vi "gugudan server.vi"() -> ()   [LabVIEW 2014]
uses:
  <vilib>/FTP/NI_FTP.lvlib
panel:
  out "불리언":bool
  in  "사용설명서":bool
  out "로그인":bool
  in  "ID":string="ID"
  in  "PW":string="PW"
  in  "명령전달":bool
  in  "address":string="ip address"
  out "명령코드":i16[](array[numeric])
  out "참 거짓":string="상태창입니다."
  out "문자열":string="q 입력시 종료 / r 입력시 종료 취소  숫자 1~3번 은 1~3시간 예약 종료 입니다."
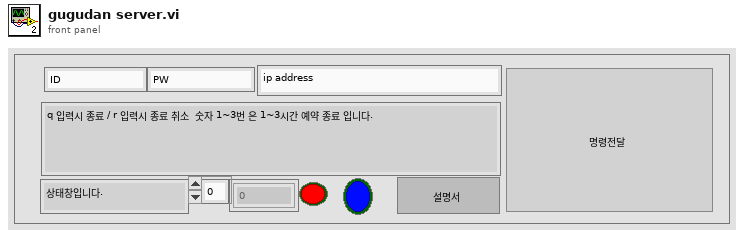
[diagram p1: front panel]
types:
  T1 = typedef "NI_FTP.lvlib/FTP Session.ctl" = refnum<k5>
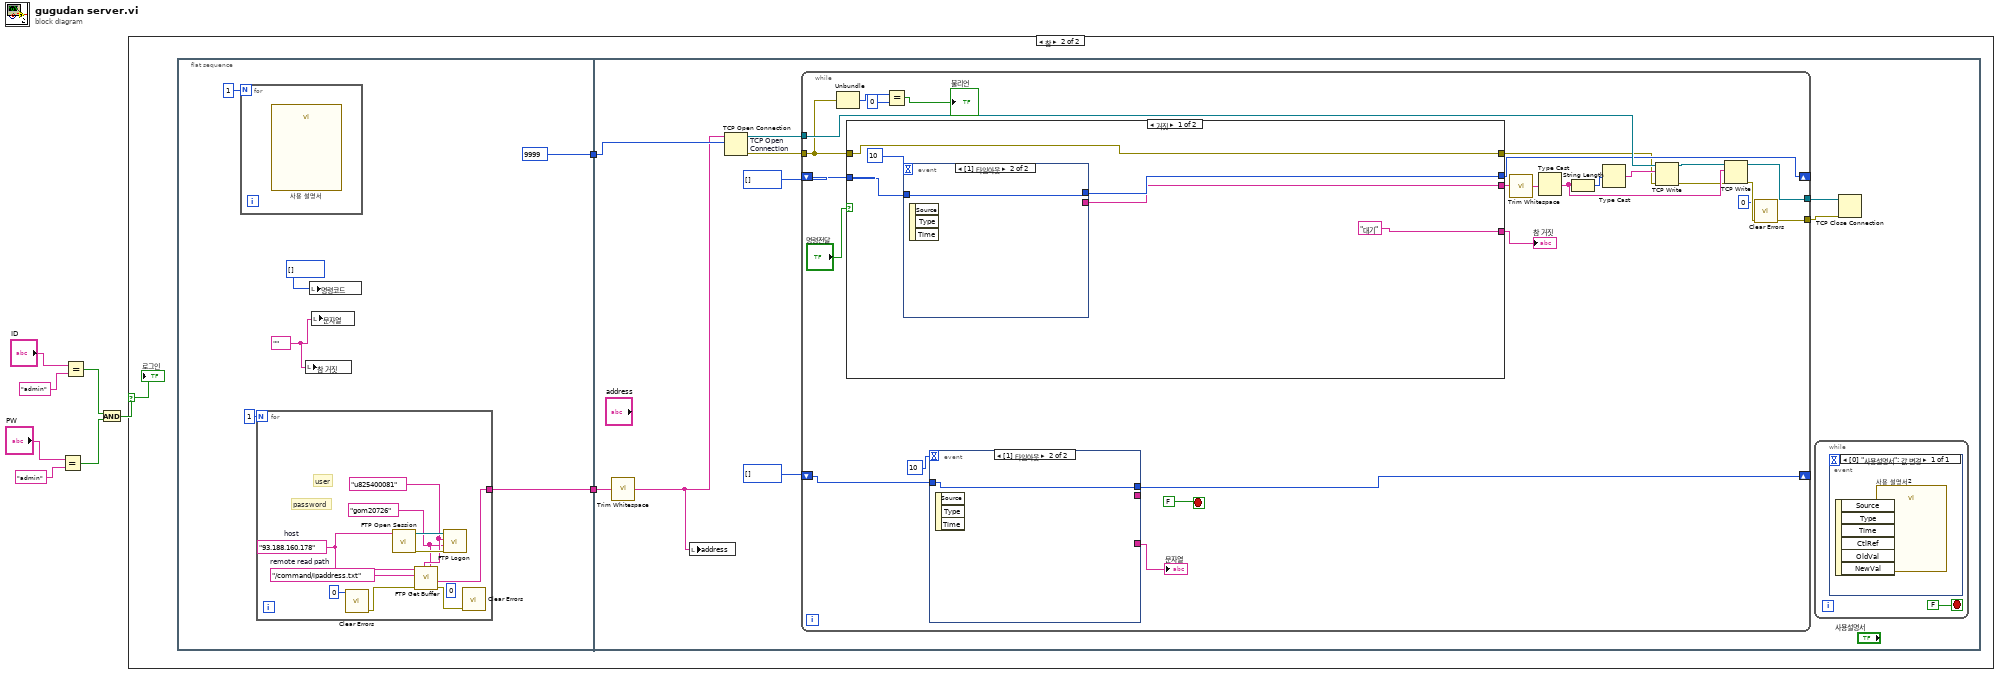
[diagram p0: block diagram]
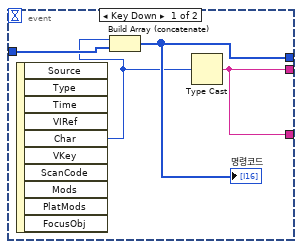
[diagram p3: hidden frame]
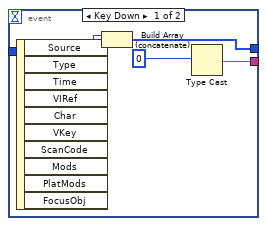
[diagram p4: hidden frame]
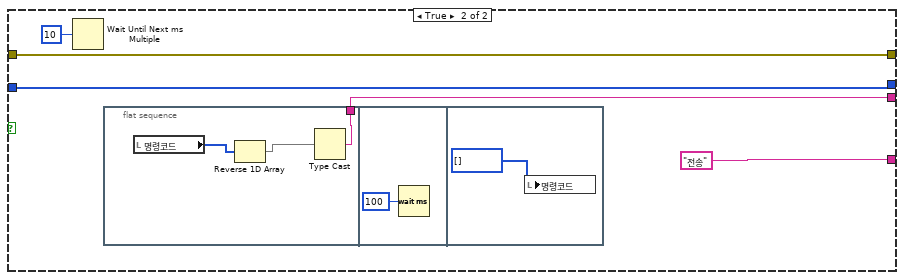
[diagram p5: hidden frame]
diagram:
  n1 = Equal?(x="PW", y="admin") -> (x = y?=w2:bool)
  n2 = Equal?(x="ID", y="admin") -> (x = y?=w3:bool)
  n3 = And(x=w3, y=w2) -> (x .and. y?=w1:bool)
  n4 = case shown="참" w1 {
    selector: w1 -> [_ w10]
    frame False {
    }
    frame True {
      n5 = flat-sequence {
        tunnel: [w12] -> w9
        tunnel: [u16 9999 ("remote port or service name")] -> w8
        tunnel: w9 -> [w29]
        tunnel: w8 -> [w28]
        frame #0 {
          w15 = ""
          n6 = for {
            N: 1 -> [_]
            n7 = call "사용 설명서"() -> ()  [unwired: 10 in, 2 out]
          }
          n8 = for {
            N: 1 -> [_]
            tunnel: [w20] -> w12
            (unwired) 0 ("specific error code to clear (0: all)")
            w23 = "gom20726"
            w24 = "u825400081"
            w21 = "/command/ipaddress.txt"  # remote read path
            w22 = "93.188.160.178"  # host
            # "user"
            # "password"
            n9 = call <vilib>:"Clear Errors.vi"("specific error code to clear (0: all)"=0) -> ("error out"=w19:errorcluster)  [unwired: 5 in, 1 out]
            n10 = call <vilib>:"FTP Open Session.vi"("address"=w22) -> ("error out"=w25:errorcluster, "ftp session"=w26:T1)  [unwired: 7 in, 2 out]
            n11 = call <vilib>:"FTP Get Buffer.vi"("password"=w23, "user"=w24, "error in (no error)"=w19, "remote path"=w21, "host"=w22) -> ("error out"=w17:errorcluster, "data"=w20:string)  [unwired: 4 in, 1 out]
            n12 = call <vilib>:"FTP Logon.vi"("error in (no error)"=w25, "password"=w23, "user"=w24, "ftp session"=w26) -> ()  [unwired: 4 in, 4 out]
            n13 = call <vilib>:"Clear Errors.vi"("error in (no error)"=w17) -> ()  [unwired: 5 in, 2 out]
          }
          n14 = local write "참 거짓"(w15) -> ()
          n15 = local write "명령코드"(i16[] []) -> ()
          n16 = local write "문자열"(w15) -> ()
        }
        frame #1 {
          n17 = call <vilib>:"Trim Whitespace.vi"("string"=w29) -> ("trimmed string"=w27:string)  [unwired: 1 in]
          n18 = local write "address"(w27) -> ()
          n19 = TCP Open Connection "TCP Open \nConnection"(address=w27, remote port or service name=w28) -> (connection ID=w35:refnum<k5>, error out=w31:errorcluster)  [unwired: 3 in]
          n20 = while {
            tunnel: w35 -> [w60]
            tunnel: [w62] -> w34
            shift-right: [w51] -> _
            shift-left: i16[] [] -> [w61]
            shift-right: [w52] -> _
            shift-left: i16[] [] -> [w53]
            tunnel: w31 -> [w40]
            tunnel: [w43] -> w30
            stop <- FALSE stop-if-true
            n21 = Unbundle(w40) -> ("code"=w39:i32)  [unwired: 2 out]
            n22 = case shown="거짓" "명령전달" {
              tunnel: w61 -> [w73 w84]
              tunnel: [w72 w84] -> w51
              tunnel: [w70 w80] -> w47
              tunnel: w40 -> [w69 w82]
              tunnel: [w69 w82] -> w50
              tunnel: ["대기" "전송"] -> w46
              frame False {
                n23 = event shown="[1] 타임아웃" {
                  selector: _ -> [_ _]
                  dyn-events: _ -> [_ _]
                  timeout: 10 -> [_ _]
                  tunnel: [w77 w79] -> w72
                  tunnel: w73 -> [w78 w79]
                  tunnel: [w75 _] -> w70
                  event Key Down {
                    n24 = event-data() -> ("Char"=w76:i16)  [unwired: 1 in, 9 out]
                    n25 = Build Array (concatenate)(w76, w78) -> (w77:i16[])
                    n26 = Type Cast(x=0) -> (*(type *) &x=w75:string)  [unwired: 1 in]
                  }
                  event Timeout {
                    n27 = event-data() -> ()  [unwired: 1 in, 3 out]
                  }
                }
              }
              frame True {
                n28 = Wait Until Next ms Multiple(millisecond multiple=u32 10) -> ()  [unwired: 1 out]
                n29 = flat-sequence {
                  tunnel: [w86] -> w80
                  frame #0 {
                    n30 = local read "명령코드"() -> (w87:i16[])
                    n31 = Reverse 1D Array(array=w87) -> (reversed array=w85:i16[])
                    n32 = Type Cast(x=w85) -> (*(type *) &x=w86:string)  [unwired: 1 in]
                  }
                  frame #1 {
                    n33 = Wait (ms)(milliseconds to wait=u32 100 ("대기 시간(ms)")) -> ()  [unwired: 1 out]
                  }
                  frame #2 {
                    n34 = local write "명령코드"(i16[] []) -> ()
                  }
                }
              }
            }
            "참 거짓" <- w46
            n35 = Equal?(x=w39, y=0) -> (x = y?=→"불리언":bool)
            n36 = event shown="[1] 타임아웃" {
              selector: _ -> [_ _]
              dyn-events: _ -> [_ _]
              timeout: 10 -> [_ _]
              tunnel: [w64 w67] -> w52
              tunnel: [w66 _] -> w54
              tunnel: [w66 _] -> _
              tunnel: w53 -> [w65 w67]
              event Key Down {
                n37 = event-data() -> ("Char"=w63:i16)  [unwired: 1 in, 9 out]
                n38 = Build Array (concatenate)(w63, w65) -> (w64:i16[])
                "명령코드" <- w64
                n39 = Type Cast(x=w63) -> (*(type *) &x=w66:string)  [unwired: 1 in]
              }
              event Timeout {
                n40 = event-data() -> ()  [unwired: 1 in, 3 out]
              }
            }
            "문자열" <- w54
            n41 = call <vilib>:"Trim Whitespace.vi"("string"=w47) -> ("trimmed string"=w48:string)  [unwired: 1 in]
            n42 = Type Cast(x=w48) -> (*(type *) &x=w56:string)  [unwired: 1 in]
            n43 = String Length(string=w56) -> (length=w57:i32)
            n44 = Type Cast(x=w57) -> (*(type *) &x=w58:string)  [unwired: 1 in]
            n45 = TCP Write(connection ID=w60, data in=w58, error in (no error)=w50) -> (connection ID out=w59:refnum<k5>, error out=w49:errorcluster)  [unwired: 1 in, 1 out]
            n46 = TCP Write(connection ID=w59, data in=w56, error in (no error)=w49) -> (connection ID out=w62:refnum<k5>, error out=w42:errorcluster)  [unwired: 1 in, 1 out]
            n47 = call <vilib>:"Clear Errors.vi"("error in (no error)"=w42, "specific error code to clear (0: all)"=0) -> ("error out"=w43:errorcluster)  [unwired: 4 in, 1 out]
          }
          n48 = while {
            stop <- FALSE stop-if-true
            n49 = event shown="[0] \"사용설명서\": 값 변경" {
              selector: _ -> [_]
              dyn-events: _ -> [_]
              timeout: _ -> [_]
              event "사용설명서": Value Change {
                n50 = event-data() -> ()  [unwired: 1 in, 6 out]
                n51 = call "사용 설명서2"() -> ()  [unwired: 10 in, 2 out]
              }
            }
          }
          n52 = TCP Close Connection(connection ID=w34, error in (no error)=w30) -> ()  [unwired: 1 in, 2 out]
        }
      }
      "로그인" <- w10
    }
  }
